vi "write status log.vi"(7 "Context ID":u32, 8 "error in":errorcluster, 9 "Action":T1, 10 "Socket Counter":u32, 11 "Context Counter":u32) -> (0 "error out":errorcluster)   [LabVIEW 2019, in "RemoteControl.ZMQ.lvlib" / "ZMQ.ContextManager.lvlib"]
uses:
  ZMQ.ContextManager.lvlib
  Typedefs/Action--enum.ctl
  <vilib>/Utility/sysdir.llb/System Directory Type.ctl
  <vilib>/Utility/file.llb/Write Delimited Spreadsheet (string).vi
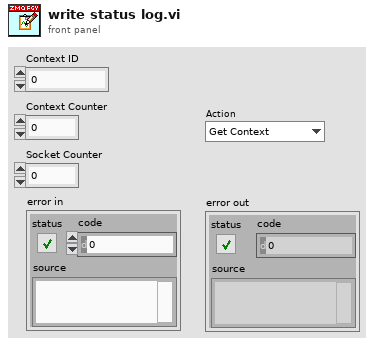
[diagram p1: front panel]
types:
  T1 = typedef "RemoteControl.ZMQ.lvlib/ZMQ.ContextManager.lvlib/Action--enum.ctl" = enum16{"Get Context", "Release Context", "Socket Opened", "Socket Closed", "Force Cleanup"}
  T2 = typedef "System Directory Type.ctl" = i32
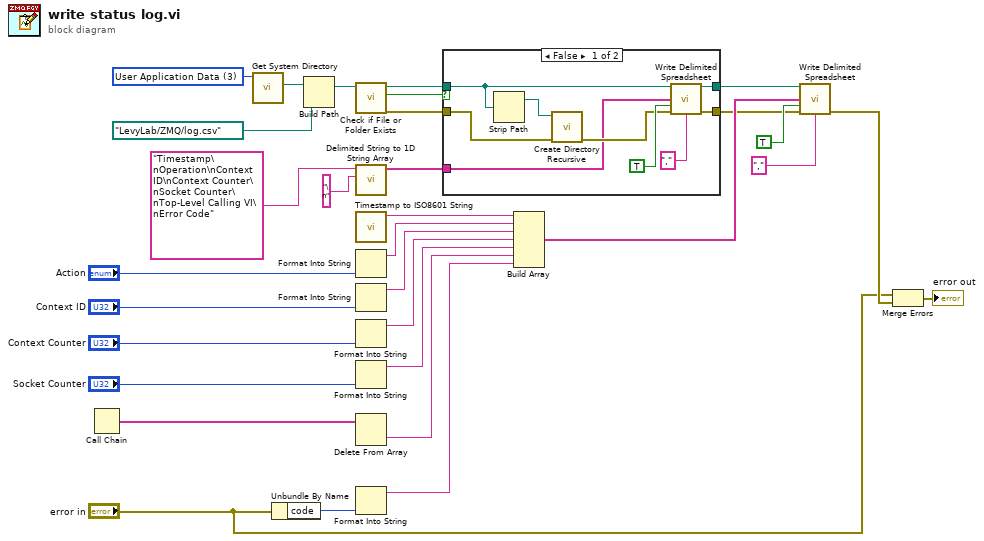
[diagram p0: block diagram]
diagram:
  w30 = T2 3 items=["User Home"=0, "User Desktop"=1, "User Documents"=2, "User Application Data"=3, "User Preferences"=4, "User Temporary"=5, "Public Documents"=6, "Public Application Data"=7, "Public Preferences"=8, "Public Cache"=13, "System Core Libraries"=9, "System Installed Libraries"=10, "Application Files"=11, "Boot Volume Root"=12] ("system directory type")
  n1 = Call Chain() -> (call chain=w9:string[])
  n2 = call <vilib>:"Get System Directory.vi"("system directory type"=w30) -> ("system directory"=w29:path)  [unwired: 10 in]
  n3 = Unbundle By Name("error in") -> ("code"=w17:i32)
  n4 = Build Path(base path=w29, name or relative path=path "LevyLab/ZMQ/log.csv") -> (appended path=w27:path)
  n5 = call <vilib>:"Check if File or Folder Exists.vi"("path"=w27) -> ("error out"=w18:errorcluster, "file or folder exists?"=w25:bool, "dup path"=w26:path)  [unwired: 8 in]
  n6 = call <vilib>:"Delimited String to 1D String Array.vi"("delimiter"="\n", "delimited string"="Timestamp\nOperation\nContext ID\nContext Counter\nSocket Counter\nTop-Level Calling VI\nError Code") -> ("string array"=w28:string[])  [unwired: 9 in]
  n7 = call <vilib>:"Timestamp to ISO8601 String.vi"() -> ("ISO8601 String"=w24:string)  [unwired: 11 in]
  n8 = Format Into String("Action") -> (resulting string=w2:string)  [unwired: 3 in, 1 out]
  n9 = Format Into String("Context ID") -> (resulting string=w3:string)  [unwired: 3 in, 1 out]
  n10 = Format Into String("Context Counter") -> (resulting string=w4:string)  [unwired: 3 in, 1 out]
  n11 = Format Into String("Socket Counter") -> (resulting string=w6:string)  [unwired: 3 in, 1 out]
  n12 = Delete From Array(array=w9) -> (deleted portion=w10:string)  [unwired: 2 in, 1 out]
  n13 = Format Into String(w17) -> (resulting string=w16:string)  [unwired: 3 in, 1 out]
  n14 = case shown="False" w25 {
    tunnel: w28 -> [w32 _]
    tunnel: w26 -> [w37 w41]
    tunnel: [w39 w41] -> w21
    tunnel: [w38 w42] -> w19
    tunnel: w18 -> [w34 w42]
    frame False {
      n15 = Strip Path(path=w37) -> (stripped path=w36:path)  [unwired: 1 out]
      n16 = call <vilib>:"Create Directory Recursive.vi"("error in (no error)"=w34, "directory"=w36) -> ("error out"=w33:errorcluster)  [unwired: 3 in, 2 out]
      n17 = call-poly <vilib>:"Write Delimited Spreadsheet.vi"("file path (dialog if empty)"=w37, "1D data"=w32, "append to file? (new file:F)"=TRUE, "error in (no error)"=w33, "delimiter (\\t)"="," ("delimiter (\\t)")) -> ("new file path (Not A Path if cancelled)"=w39:path, "error out"=w38:errorcluster)  [unwired: 9 in]
    }
    frame True {
    }
  }
  n18 = Build Array(w24, w2, w3, w4, w6, w10, w16) -> (w20:string[])
  n19 = call-poly <vilib>:"Write Delimited Spreadsheet.vi"("file path (dialog if empty)"=w21, "1D data"=w20, "append to file? (new file:F)"=TRUE, "error in (no error)"=w19, "delimiter (\\t)"="," ("delimiter (\\t)")) -> ("error out"=w13:errorcluster)  [unwired: 9 in, 1 out]
  n20 = Merge Errors("error in", w13) -> (→"error out":errorcluster)
